vi "Stop Core.vi"(10 "final error code":i32, 11 "Connection in":refnum<class "Connection.lvclass">) -> (3 "Connection out":refnum<class "Connection.lvclass">)   [LabVIEW 2022 SP3, in "Connection.lvlib" / "Connection.lvclass"]
doc: "(<B>Filename</B>: Actor Framework.lvlib:Actor.lvclass:Stop Core.vi)\n\nDefines what the actor does before it stops. Use the <B>final error code</B> input to determine whether the actor shut down in response to an error.\n\nBy default, this method does nothing. A descendant class may override it to define behavior, such as shutting down any processes the actor initiated in its override of the Actor Core method."
uses:
  Connection.lvclass
  C:/Program Files (x86)/National Instruments/LabVIEW 2022/vi.lib/ActorFramework/Actor/Actor.lvclass
  <vilib>/ActorFramework/Actor/Actor.lvclass/Actor.ctl
  Connection.lvclass/Connection.ctl
  CallerMessage Messages/ConnectionDied Msg/ConnectionDied Msg.lvclass/ConnectionDied Msg.ctl
  <vilib>/ActorFramework/Message Enqueuer/Message Enqueuer.lvclass/Message Enqueuer.ctl
  <vilib>/ActorFramework/Message Enqueuer/Enqueue.vi
  CallerMessage Messages/ConnectionDied Msg/ConnectionDied Msg.lvclass
  C:/Program Files (x86)/National Instruments/LabVIEW 2022/vi.lib/ActorFramework/Message/Message.lvclass
  <vilib>/ActorFramework/Message Priority Queue/Priority Enqueue.vi
  LoggingActor/Source/LoggingActor/LoggingActor/LoggingActor.lvclass
  <vilib>/ActorFramework/Actor/Actor.lvclass
  TcpSocket/Source/TcpSocket/Connection/Connection.lvclass
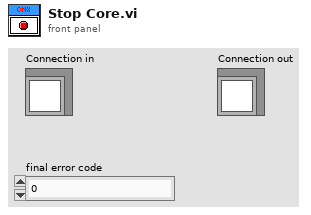
[diagram p1: front panel]
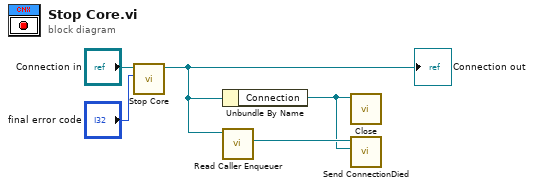
[diagram p0: block diagram]
diagram:
  n1 = call-parent "Stop Core.vi"("final error code"="final error code", "LoggingActor in"="Connection in") -> ("LoggingActor out"=w2:refnum<class "Connection.lvclass">)  [unwired: 9 in]
  "Connection out" <- w2
  n2 = Unbundle By Name(w2) -> ("Connection"=w1:refnum<class "Connection.lvclass">)
  n3 = call <vilib>:"Read Caller Enqueuer.vi"("Actor"=w2) -> ("Caller Enqueuer"=w3:refnum<class "Message Enqueuer.lvclass">)  [unwired: 10 in]
  n4 = call-dynamic "Close.vi"("Connection"=w1) -> ()  [unwired: 10 in, 1 out]
  n5 = call "Send ConnectionDied.vi"("Connection"=w1, "Message Enqueuer"=w3) -> ()  [unwired: 8 in, 2 out]
